vi "GetTUIDFromDB.vi"(8 "error in":errorcluster caption="错误输入（无错误）", 9 "PartNumber":string, 11 "DeviceType":string) -> (0 "error out":errorcluster caption="错误输出", 1 "Empty？":bool, 2 "Certid":string, 3 "TUID":string)   [LabVIEW 2013]
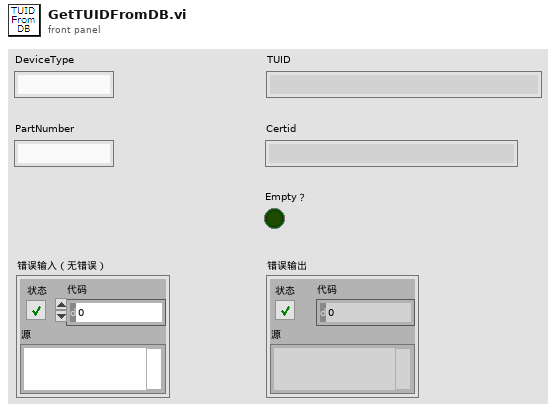
[diagram p1: front panel]
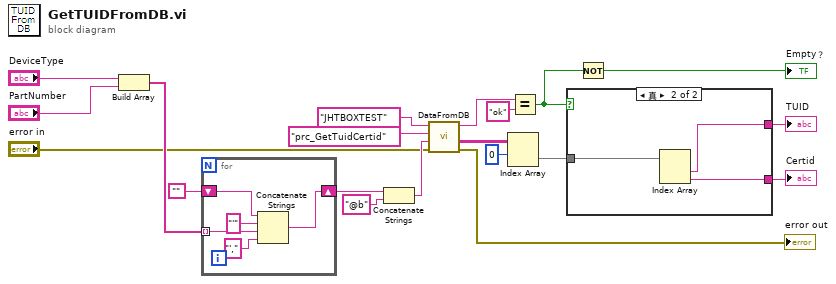
[diagram p0: block diagram]
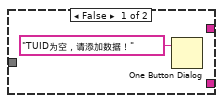
[diagram p2: hidden frame]
diagram:
  n1 = Build Array("DeviceType", "PartNumber") -> (w17:string[])
  n2 = for {
    shift-right: [w24] -> w16
    shift-left: "" -> [w25]
    tunnel: w17 -> [w23] mode=indexing
    n3 = Concatenate Strings(w25, "'", w23, "',") -> (w24:string)
  }
  n4 = Concatenate Strings(w16, "@b") -> (w14:string)
  n5 = call "DataFromDB.vi"("error in"="error in", "all string"=w14, "Procedure name"="prc_GetTuidCertid", "DSN name"="JHTBOXTEST") -> ("error out"=→"error out":errorcluster, "DataOut"=w8:string[][], "Result"=w10:string)  [unwired: 5 in]
  n6 = Index Array(array=w8, index (row)=0 ("索引 (行)")) -> (element=w6:string[])  [unwired: 1 in]
  n7 = Equal?(x=w10, y="ok" ("DSN name")) -> (x = y?=w1:bool)
  n8 = case shown="真" w1 {
    tunnel: w6 -> [_ w29]
    tunnel: [_ w28] -> w5
    tunnel: [_ w27] -> w4
    frame False {
      n9 = One Button Dialog(message="TUID为空，请添加数据！" ("消息")) -> ()  [unwired: 1 in, 1 out]
    }
    frame True {
      n10 = Index Array(array=w29) -> (element #1=w28:string, element #2=w27:string)  [unwired: 2 in]
    }
  }
  "TUID" <- w5
  "Certid" <- w4
  n11 = Not(x=w1) -> (.not. x?=→"Empty？":bool)
